vi "CSM - Global Log Error Handler.vi"(6 "Clear Error? (T)":bool=TRUE, 7 "Place (\"\" to Use VI's Name)":string, 8 "Error In":errorcluster caption="error in (no error)") -> (0 "error out":errorcluster)   [LabVIEW 2017, in "Communicable State Machine.lvlib"]
doc: "CSM error handling function. If an error occurs, the error information is published via the CSM Global Log. This allows error information occurring outside the CSM framework to be recorded in the global log.\n\n-- <b>Controls</b> --\n- <b>Place (\"\" to Use VI's Name)</b>: Marks the location where the error occurred, which by default uses the name of the calling VI.\n- <b>Clear Error? (T)</b>: Whether to clear the error. The default is TRUE, which specifies to clear the error. The error is cleared after passing through this VI."
uses:
  Communicable State Machine.lvlib
  _Support/Typedef/_CSM_GlobalLog_MSG.ctl
  _Support/Typedef/_CSM_Response Source Message.ctl
  _Support/Typedef/_CSM_GlobalLog_MSG_TYPE.ctl
  CSM - Make String Arguments Safe.vi
  _Support/GlobalEvent/GEvt-Convert Filter Rules - v1.2.vi
  _Support/ChangeFlag/FlagInstance-GEvt Filter.vi
  _Support/ChangeFlag/FlagInstance-GEvt Refs.vi
  CSM - Keywords.vi
  _Support/ChangeFlag/ChangeFlag-Read.vi
  _Support/GlobalEvent/LogFilter/LogFilter - Check.vi
  _Support/GlobalEvent/LogFilter/SettingVIs/Set Periodic Log Filter.vi
  _Support/GlobalEvent/LogFilter/SettingVIs/Set CSM Broadcast Filter.vi
  _Support/GlobalEvent/LogFilter/SettingVIs/Set CSM StateType Filter.vi
  _Support/GlobalEvent/LogFilter/SettingVIs/Set Global StateType Filter.vi
  _Support/GlobalEvent/LogFilter/SettingVIs/Set CSM State Filter.vi
  _Support/GlobalEvent/LogFilter/SettingVIs/Set CSM LogType Filter.vi
  _Support/GlobalEvent/LogFilter/SettingVIs/Set Global Broadcast Filter.vi
  _Support/GlobalEvent/LogFilter/SettingVIs/Set Global State Filter.vi
  _Support/GlobalEvent/LogFilter/SettingVIs/Set Global LogType Filter.vi
  _Support/GlobalEvent/LogFilter/SettingVIs/Set Global CSM Filter.vi
  _Support/GlobalEvent/FGV-GEvt Filter Rules(lvlibp).vi
  _Support/ChangeFlag/ChangeFlagDB.vi
  _Support/GlobalEvent/GEvt-Valid Subscribers.vi
  _Support/GlobalEvent/FGV-GlobalEventQueues(lvlibp).vi
  _Support/GlobalEvent/FGV-GlobalEventRef(lvlibp).vi
  _Support/GlobalEvent/LogFilter/LogFilter.lvclass
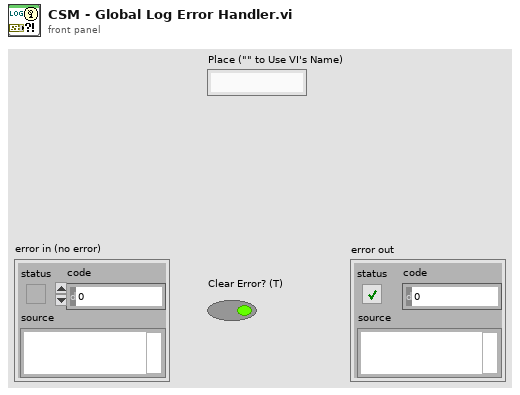
[diagram p1: front panel]
types:
  T1 = typedef "Communicable State Machine.lvlib/_CSM_GlobalLog_MSG_TYPE.ctl" = enum16{"User Log", "State Change", "Status", "Interrupt", "Register", "Unregister", "Error Log", "Module Created", "Module Destroyed", "Async Message", "No-Rep Async Message", "Sync Message", "AsyncMsg Complete", "SyncMsg Complete"}
  T2 = typedef "Communicable State Machine.lvlib/_CSM_GlobalLog_MSG.ctl" = cluster{"Name (\"\" to Use UUID)":string, "Current State":string, "Arguments":string, "Source Message":T3, "Source Module":string, "Complete(T)/Start(F)":bool, "LogType":T1, "Time Stamp":timestamp}
  T3 = typedef "Communicable State Machine.lvlib/_CSM_Response Source Message.ctl" = cluster{"‘State":string, "’Arguments":string, "’Error":errorcluster}
  T4 = typedef "Communicable State Machine.lvlib/GEvt-Refs.ctl" = cluster{"Event":refnum<user-event>, "Queues":refnum<queue>[], "Valid":bool}
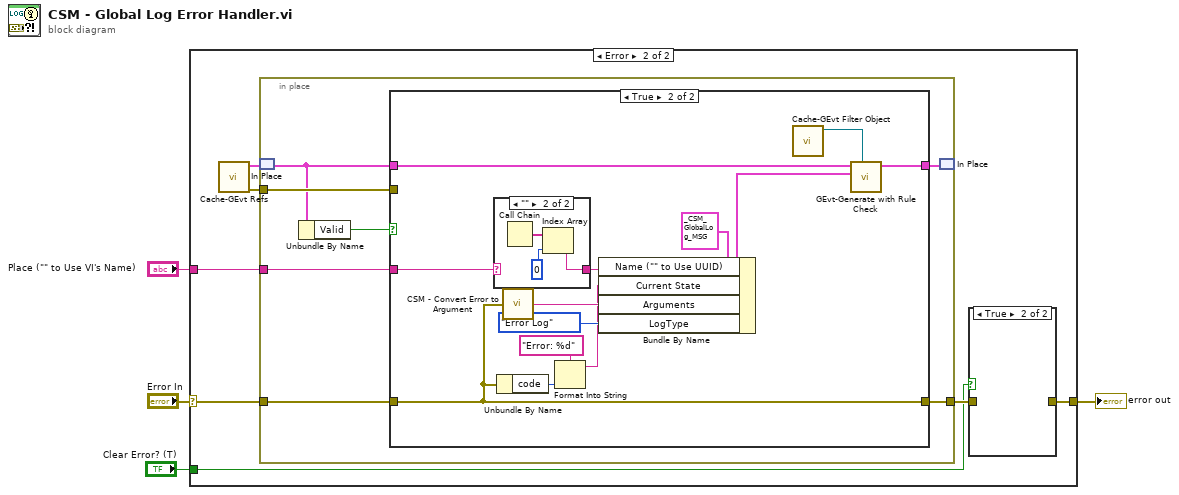
[diagram p0: block diagram]
diagram:
  n1 = case shown="Error" "Error In" {
    selector: "Error In" -> [w5 w11]
    tunnel: [w5 w9] -> w4
    tunnel: "Place (\"\" to Use VI's Name)" -> [_ w12]
    tunnel: "Clear Error? (T)" -> [_ w8]
    frame No Error {
    }
    frame Error {
      n2 = call "Cache-GEvt Refs.vi"() -> ("error out"=w6:errorcluster, "CSM Global Log Ref"=w7:T4)  [unwired: 10 in]
      n3 = in-place {
        in-place-border: w12 -> [w19]
        in-place-border: w6 -> [w18]
        in-place-border: w11 -> [w17]
        in-place-border: [w16] -> w10
        n4 = in-place-match #1(w7) -> (w14:T4)
        n5 = Unbundle By Name(w14) -> ("Valid"=w15:bool)
        n6 = case shown="True" w15 {
          tunnel: w14 -> [w22 w25]
          tunnel: w19 -> [_ w29]
          tunnel: [w22 w24] -> w20
          tunnel: w18 -> [_ _]
          tunnel: w17 -> [w21 w27]
          tunnel: [w21 w27] -> w16
          frame False {
          }
          frame True {
            n7 = case shown="\"\"" w29 {
              selector: w29 -> [w36 _]
              tunnel: [w36 w37] -> w28
              frame Default {
              }
              frame "" {
                n8 = Call Chain() -> (call chain=w38:string[])
                n9 = Index Array(array=w38, index=0 ("Index")) -> (element=w37:string)
              }
            }
            n10 = Unbundle By Name(w27) -> ("code"=w32:i32)
            n11 = call "CSM - Convert Error to Argument.vi"("Error"=w27) -> ("Argument"=w33:string)  [unwired: 4 in]
            n12 = Format Into String(format string="Error: %d", w32) -> (resulting string=w30:string)  [unwired: 2 in, 1 out]
            n13 = Bundle By Name(cluster=T2 {"Name (\"\" to Use UUID)"="", "Current State"="", "Arguments"="", "Source Message"={"‘State"="", "’Arguments"="", "’Error"={"status"=FALSE, "code"=0, "source"=""}}, "Source Module"="", "Complete(T)/Start(F)"=FALSE, "LogType"=enum."User Log", "Time Stamp"=timestamp(0 s since 1904-01-01)} ("event data"), "Name (\"\" to Use UUID)"=w28, "Current State"=w30, "Arguments"=w33, "LogType"=_CSM_GlobalLog_MSG_TYPE."Error Log" ("Type")) -> (w26:T2)
            n14 = call "Cache-GEvt Filter Object.vi"() -> ("CSM:LogFilter.lvclass"=w23:refnum<class "LogFilter.lvclass">)  [unwired: 11 in]
            n15 = call "GEvt-Generate with Rule Check.vi"("LogFilter In"=w23, "Event Data"=w26, "CSM Global Log Event In"=w25) -> ("CSM Global Log Event Out"=w24:T4)  [unwired: 8 in]
          }
        }
        n16 = in-place-match #1(w20) -> ()  [unwired: 1 out]
      }
      n17 = case shown="True" w8 {
        tunnel: w10 -> [w13 _]
        tunnel: [w13 _] -> w9
        frame False {
        }
        frame True {
        }
      }
    }
  }
  "error out" <- w4
